vi "pixxelMultiControl.vi"(4 "u16":u16, 5 "baseAddress":string, 7 "PIXXELaction":T1=enum."close", 8 "error in (no error)":errorcluster, 11 "AnzPois":i32) -> (0 "error out":errorcluster, 3 "activeTCP":bool[](array[boolean]))   [LabVIEW 2014]
uses:
  typeDefs/pixxelMultiAction.ctl
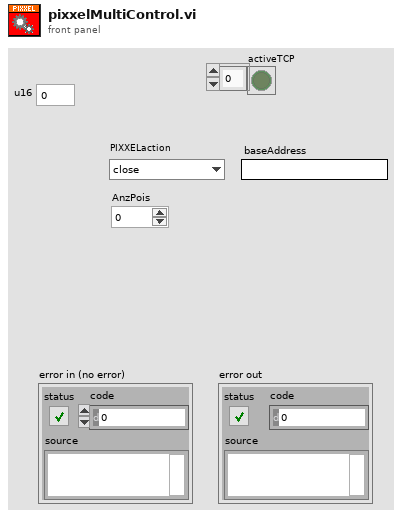
[diagram p1: front panel]
types:
  T1 = typedef "pixxelMultiAction.ctl" = enum16{"init", "initAll", "initMissing", "watchdog", "black", "close", "startProg", "pauseProg", "stopProg", "jumpTo"}
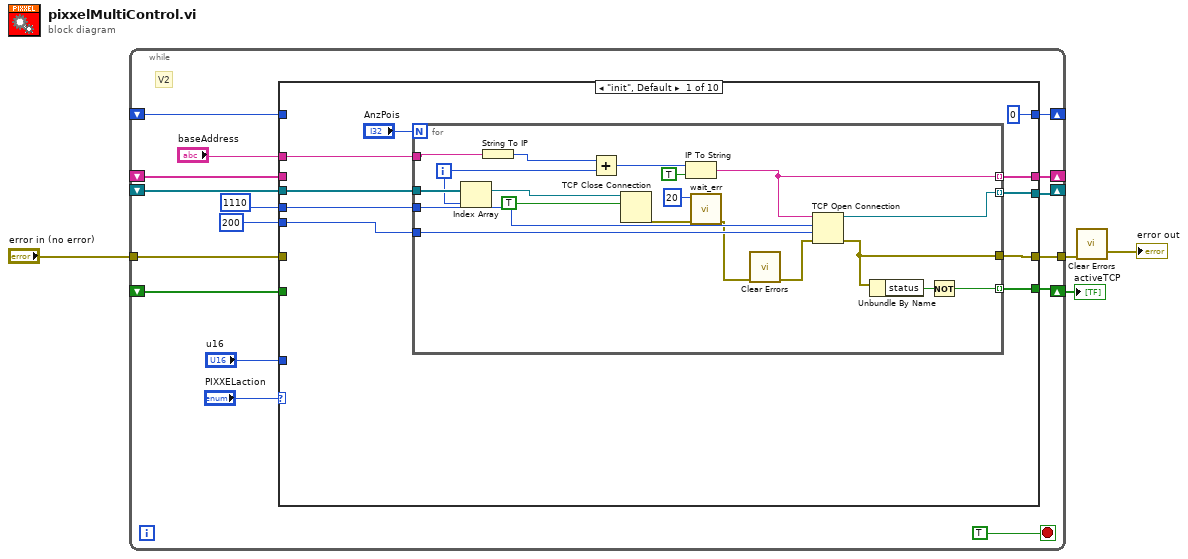
[diagram p0: block diagram]
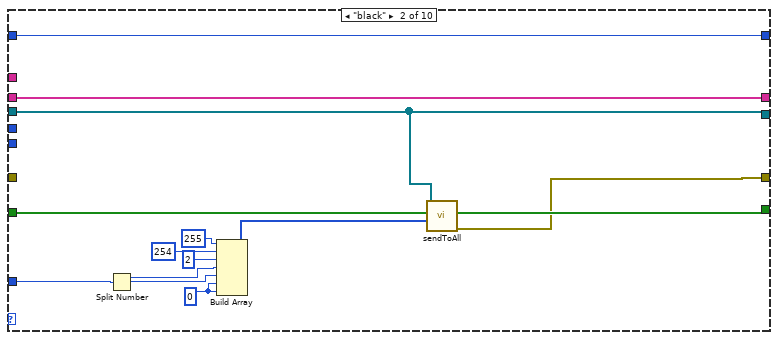
[diagram p2: hidden frame]
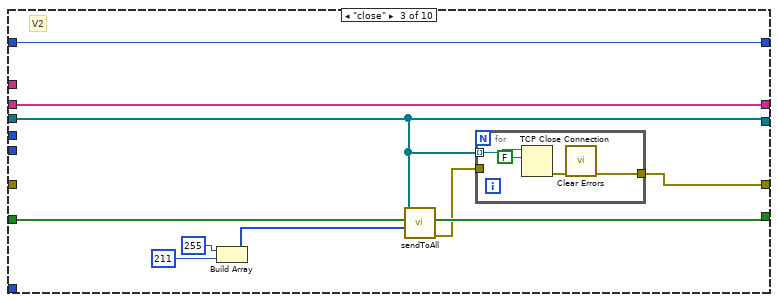
[diagram p3: hidden frame]
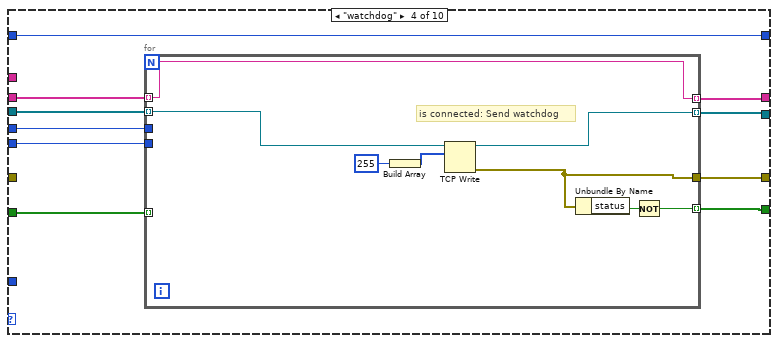
[diagram p4: hidden frame]
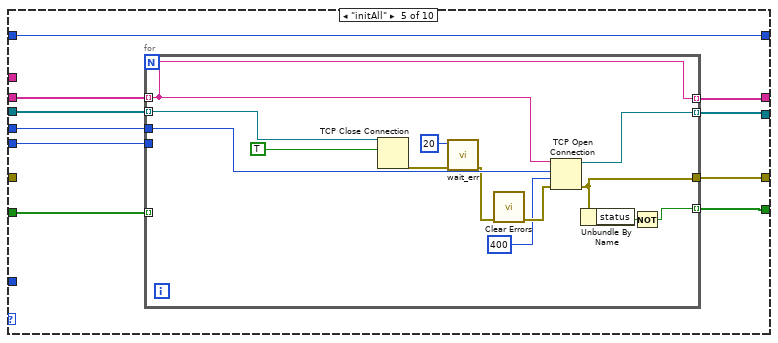
[diagram p5: hidden frame]
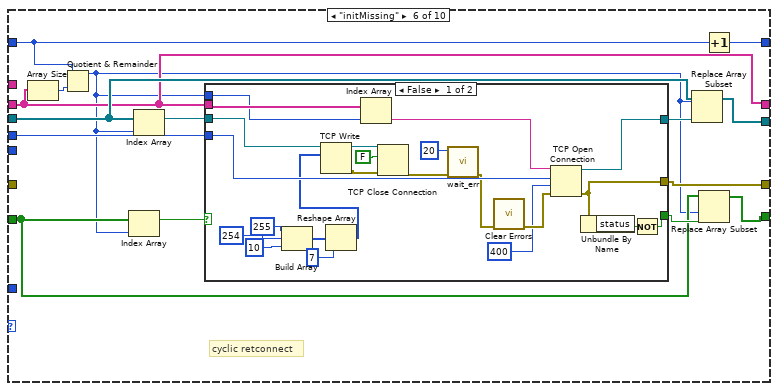
[diagram p6: hidden frame]
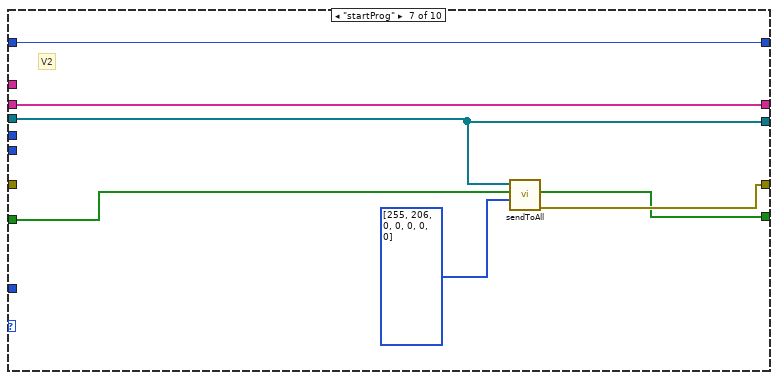
[diagram p8: hidden frame]
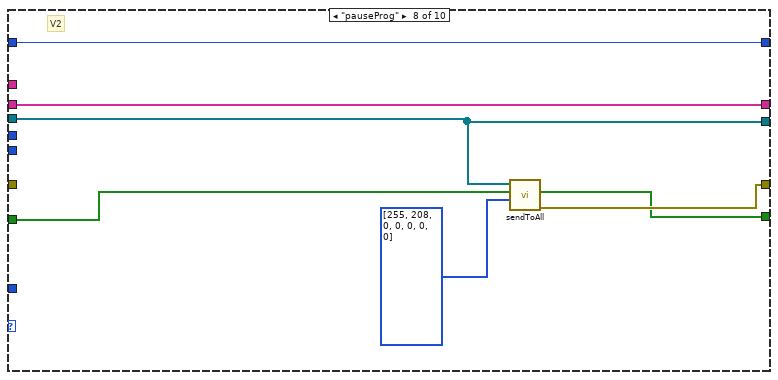
[diagram p9: hidden frame]
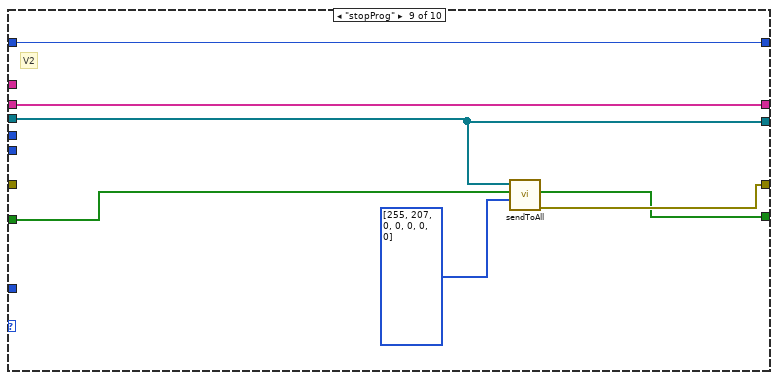
[diagram p10: hidden frame]
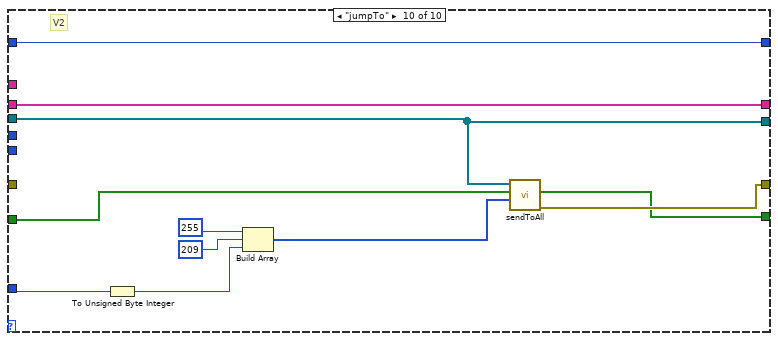
[diagram p11: hidden frame]
diagram:
  n1 = while {
    shift-right: [w15] -> _
    shift-left: _ -> [w16]
    tunnel: [w18] -> w4
    tunnel: "error in (no error)" -> [w17]
    shift-right: [w12] -> _
    shift-left: _ -> [w11]
    shift-right: [w8] -> w2
    shift-left: _ -> [w7]
    shift-right: [w5] -> _
    shift-left: _ -> [w6]
    stop <- TRUE stop-if-true
    # "V2"
    n2 = case shown="\"init\", Default" "PIXXELaction" {
      tunnel: [w22 w52 w66 w80 w98 w132 w165 w172 w179 w190] -> w18
      tunnel: w17 -> [_ _ _ _ _ _ _ _ _ _]
      tunnel: w16 -> [w30 w55 w67 w87 w105 w129 w161 w168 w175 w187]
      tunnel: [w25 w55 w67 w86 w104 w127 w161 w168 w175 w187] -> w15
      tunnel: u16 1110 ("remote port or service name") -> [w29 _ _ w83 w101 w133 _ _ _ _]
      tunnel: 200 ("timeout ms (60000)") -> [w28 _ _ w82 w100 _ _ _ _ _]
      tunnel: [w27 w60 w71 w79 w97 w122 w164 w171 w178 w189] -> w12
      tunnel: w11 -> [_ w60 w71 w84 w102 w122 w164 w171 w178 w189]
      tunnel: "u16" -> [_ w57 _ _ _ _ _ _ _ w183]
      tunnel: "baseAddress" -> [w24 _ _ _ _ _ _ _ _ _]
      tunnel: [w23 w53 w69 w81 w99 w124 w160 w167 w174 w186] -> w8
      tunnel: w7 -> [_ w54 w70 w85 w103 w125 w162 w169 w176 w188]
      tunnel: w6 -> [_ w50 w64 w78 w96 w120 w159 w166 w173 w180]
      tunnel: [0 w50 w64 w78 w96 w123 w159 w166 w173 w180] -> w5
      frame "init", Default {
        n3 = for {
          N: "AnzPois" -> [_]
          tunnel: w30 -> [w49]
          tunnel: w29 -> [w46]
          tunnel: w28 -> [w45]
          tunnel: [w39] -> w27 mode=indexing
          tunnel: [w41] -> w25 mode=indexing
          tunnel: w24 -> [w37]
          tunnel: [w34] -> w23 mode=indexing
          tunnel: [w33] -> w22
          i -> [w31]
          n4 = Index Array(array=w49, index=w31) -> (element=w32:refnum<k5>)
          n5 = String To IP(1:w37) -> (0:w36:u32)
          n6 = Add(x=w36, y=w31) -> (x+y=w40:u32)
          n7 = TCP Close Connection(connection ID=w32, abort (F)=TRUE) -> (error out=w48:errorcluster)  [unwired: 1 in, 1 out]
          n8 = IP To String(1:TRUE ("dot notation? (F)"), 2:w40) -> (0:w39:string)
          n9 = call <userlib>:"wait_err.vi"("error in (no error)"=w48, "milliseconds to wait"=u32 20) -> ("error out"=w44:errorcluster)  [unwired: 9 in]
          n10 = call <vilib>:"Clear Errors.vi"("error in (no error)"=w44) -> ("error out"=w43:errorcluster)  [unwired: 5 in, 1 out]
          n11 = TCP Open Connection(address=w39, remote port or service name=w46, timeout ms (60000)=w45, error in (no error)=w43) -> (connection ID=w41:refnum<k5>, error out=w33:errorcluster)  [unwired: 1 in]
          n12 = Unbundle By Name(w33) -> ("status"=w35:bool)
          n13 = Not(x=w35) -> (.not. x?=w34:bool)
        }
      }
      frame "black" {
        w56 = u8 0 ("element")
        n14 = Split Number(x=w57) -> (hi(x)=w59:u8, lo(x)=w58:u8)
        n15 = Build Array(u8 255 ("element"), u8 254 ("element"), u8 2 ("element"), w59, w58, w56, w56) -> (w51:u8[])
        n16 = call "sendToAll.vi"("Data"=w51, "TCPok"=w54, "TCPconns"=w55) -> ("error out"=w52:errorcluster, "activeTCP"=w53:bool[])  [unwired: 7 in]
      }
      frame "close" {
        # "V2"
        n17 = Build Array(u8 255 ("element"), u8 211 ("element")) -> (w68:u8[])
        n18 = call "sendToAll.vi"("Data"=w68, "TCPok"=w70, "TCPconns"=w67) -> ("error out"=w65:errorcluster, "activeTCP"=w69:bool[])  [unwired: 7 in]
        n19 = for {
          tunnel: w67 -> [w76] mode=indexing
          tunnel: [w74] -> w66
          tunnel: w65 -> [_]
          n20 = TCP Close Connection(connection ID=w76, abort (F)=FALSE) -> (error out=w75:errorcluster)  [unwired: 1 in, 1 out]
          n21 = call <vilib>:"Clear Errors.vi"("error in (no error)"=w75) -> ("error out"=w74:errorcluster)  [unwired: 5 in, 1 out]
        }
      }
      frame "watchdog" {
        n22 = for {
          tunnel: w87 -> [w95] mode=indexing
          tunnel: [w94] -> w86 mode=indexing
          tunnel: w85 -> [_] mode=indexing
          tunnel: w84 -> [w91] mode=indexing
          tunnel: w83 -> [_]
          tunnel: w82 -> [_]
          tunnel: [w93] -> w80
          tunnel: [w92] -> w81 mode=indexing
          tunnel: [w91] -> w79 mode=indexing
          # "is connected: Send watchdog"
          n23 = Build Array(u8 255 ("element")) -> (w89:u8[])
          n24 = TCP Write(connection ID=w95, data in=w89) -> (connection ID out=w94:refnum<k5>, error out=w93:errorcluster)  [unwired: 2 in, 1 out]
          n25 = Unbundle By Name(w93) -> ("status"=w88:bool)
          n26 = Not(x=w88) -> (.not. x?=w92:bool)
        }
      }
      frame "initAll" {
        n27 = for {
          tunnel: w105 -> [w118] mode=indexing
          tunnel: [w117] -> w104 mode=indexing
          tunnel: w103 -> [_] mode=indexing
          tunnel: w102 -> [w113] mode=indexing
          tunnel: w101 -> [w116]
          tunnel: w100 -> [_]
          tunnel: [w115] -> w98
          tunnel: [w114] -> w99 mode=indexing
          tunnel: [w113] -> w97 mode=indexing
          n28 = TCP Close Connection(connection ID=w118, abort (F)=TRUE) -> (error out=w109:errorcluster)  [unwired: 1 in, 1 out]
          n29 = call <userlib>:"wait_err.vi"("error in (no error)"=w109, "milliseconds to wait"=u32 20) -> ("error out"=w111:errorcluster)  [unwired: 9 in]
          n30 = call <vilib>:"Clear Errors.vi"("error in (no error)"=w111) -> ("error out"=w112:errorcluster)  [unwired: 5 in, 1 out]
          n31 = TCP Open Connection(address=w113, remote port or service name=w116, timeout ms (60000)=400, error in (no error)=w112) -> (connection ID=w117:refnum<k5>, error out=w115:errorcluster)  [unwired: 1 in]
          n32 = Unbundle By Name(w115) -> ("status"=w107:bool)
          n33 = Not(x=w107) -> (.not. x?=w114:bool)
        }
      }
      frame "initMissing" {
        # "cyclic retconnect"
        n34 = Array Size(array=w122) -> (size(s)=w121:i32)
        n35 = Quotient & Remainder(x=w120, y=w121) -> (x-y*floor(x/y)=w119:i32)  [unwired: 1 out]
        n36 = Index Array(array=w125, index=w119) -> (element=w130:bool)
        n37 = Index Array(array=w129, index=w119) -> (element=w131:refnum<k5>)
        n38 = case shown="False" w130 {
          selector: w130 -> [_ w157]
          tunnel: w131 -> [w139 w158]
          tunnel: [w156 w158] -> w128
          tunnel: w133 -> [w155 _]
          tunnel: [w154 _] -> w132
          tunnel: [w153 w157] -> w126
          tunnel: w122 -> [w145 _]
          tunnel: w119 -> [w143 _]
          frame False {
            n39 = Build Array(u8 255 ("element"), u8 254 ("element"), u8 10 ("element")) -> (w137:u8[])
            n40 = Reshape Array(w137, 7 ("dimension size")) -> (w135:u8[])
            n41 = TCP Write(connection ID=w139, data in=w135) -> (connection ID out=w138:refnum<k5>, error out=w134:errorcluster)  [unwired: 2 in, 1 out]
            n42 = Index Array(array=w145, index=w143) -> (element=w144:string)
            n43 = TCP Close Connection(connection ID=w138, abort (F)=FALSE, error in (no error)=w134) -> (error out=w149:errorcluster)  [unwired: 1 out]
            n44 = call <userlib>:"wait_err.vi"("error in (no error)"=w149, "milliseconds to wait"=u32 20) -> ("error out"=w151:errorcluster)  [unwired: 9 in]
            n45 = call <vilib>:"Clear Errors.vi"("error in (no error)"=w151) -> ("error out"=w152:errorcluster)  [unwired: 5 in, 1 out]
            n46 = TCP Open Connection(address=w144, remote port or service name=w155, timeout ms (60000)=400, error in (no error)=w152) -> (connection ID=w156:refnum<k5>, error out=w154:errorcluster)  [unwired: 1 in]
            n47 = Unbundle By Name(w154) -> ("status"=w147:bool)
            n48 = Not(x=w147) -> (.not. x?=w153:bool)
          }
          frame True {
          }
        }
        n49 = Replace Array Subset(array=w129, new element=w128, index=w119) -> (w127:refnum<k5>[])
        n50 = Replace Array Subset(array=w125, new element=w126, index=w119) -> (w124:bool[])
        n51 = Increment(x=w120) -> (x+1=w123:i32)
      }
      frame "startProg" {
        # "V2"
        n52 = call "sendToAll.vi"("Data"=u8[] [255, 206, 0, 0, 0, 0, 0], "TCPok"=w162, "TCPconns"=w161) -> ("error out"=w165:errorcluster, "activeTCP"=w160:bool[])  [unwired: 7 in]
      }
      frame "pauseProg" {
        # "V2"
        n53 = call "sendToAll.vi"("Data"=u8[] [255, 208, 0, 0, 0, 0, 0], "TCPok"=w169, "TCPconns"=w168) -> ("error out"=w172:errorcluster, "activeTCP"=w167:bool[])  [unwired: 7 in]
      }
      frame "stopProg" {
        # "V2"
        n54 = call "sendToAll.vi"("Data"=u8[] [255, 207, 0, 0, 0, 0, 0], "TCPok"=w176, "TCPconns"=w175) -> ("error out"=w179:errorcluster, "activeTCP"=w174:bool[])  [unwired: 7 in]
      }
      frame "jumpTo" {
        # "V2"
        n55 = To Unsigned Byte Integer(number=w183) -> (unsigned 8bit integer=w182:u8)
        n56 = Build Array(u8 255 ("element"), u8 209 ("element"), w182) -> (w181:u8[])
        n57 = call "sendToAll.vi"("Data"=w181, "TCPok"=w188, "TCPconns"=w187) -> ("error out"=w190:errorcluster, "activeTCP"=w186:bool[])  [unwired: 7 in]
      }
    }
  }
  "activeTCP" <- w2
  n58 = call <vilib>:"Clear Errors.vi"("error in (no error)"=w4) -> ("error out"=→"error out":errorcluster)  [unwired: 5 in, 1 out]
